vi "FP PC main.vi"() -> ()   [LabVIEW 2014]
panel:
  in  "Tab Control":enum32{"Front Page", "Mission Definition"}(tab)
  in  "Chase?":bool
  in  "stop":bool
  in  "Tug letter":string="T"
  out "UDP Time Out?":bool
  out "Blink":bool
  out "error IO":errorcluster
  out "GPS":cluster{"X pos":i32, "Y pos":i32, "Heading":dbl}
  out "Grid Image":T1(plugin-control)
  in  "Pool image\nfile name":string="leds in brightfield cropped.bmp"
  in  "Boat image\nfile name":string="large boat image.png"
  out "Occupancy Grid":u32[][](array[numeric])
  out "Buoy locations":cluster{"regular expression":string, i32, i32}[](array[cluster])
  out "GPS?":bool
  in  "Mission #":enum16{"1", "2", "3"}(ring)
  in  "Use mission?":bool
  in  "MDF Control":T2(array[cluster])=[{"Type"=enum."Start", "X"=100, "Y"=100, "Speed"=10, "Behaviors"=enum."Open Water Transit"}, {"Type"=enum."Waypoint", "X"=449, "Y"=569, "Speed"=4, "Behaviors"=enum."Open Water Transit"}, {"Type"=enum."Waypoint", "X"=803, "Y"=515, "Speed"=4, "Behaviors"=enum."Open Water Transit"}, {"Type"=enum."Waypoint", "X"=911, "Y"=689, "Speed"=4, "Behaviors"=enum."Open Water Transit"}, {"Type"=enum."Waypoint", "X"=755, "Y"=881, "Speed"=4, "Behaviors"=enum."Open Water Transit"}, {"Type"=enum."End", "X"=0, "Y"=0, "Speed"=0, "Behaviors"=enum."Open Water Transit"}]
  out "MDF To Send":T2(array[cluster])=[{"Type"=enum."Start", "X"=100, "Y"=100, "Speed"=10, "Behaviors"=enum."Open Water Transit"}, {"Type"=enum."Waypoint", "X"=449, "Y"=569, "Speed"=4, "Behaviors"=enum."Open Water Transit"}, {"Type"=enum."Waypoint", "X"=803, "Y"=515, "Speed"=4, "Behaviors"=enum."Open Water Transit"}, {"Type"=enum."Waypoint", "X"=911, "Y"=689, "Speed"=4, "Behaviors"=enum."Open Water Transit"}, {"Type"=enum."Waypoint", "X"=755, "Y"=881, "Speed"=4, "Behaviors"=enum."Open Water Transit"}, {"Type"=enum."End", "X"=0, "Y"=0, "Speed"=0, "Behaviors"=enum."Open Water Transit"}]
  # "This page is used to plan the mission.  The MDF, Mission Definition File, control below is used for that purpose.\n\n*  Each mission must begin with a record of type \"Start\" and end with a record of type \"End\"\n*  For the \"Start\" and \"End\" records the remaining entries have no impact.\n*  For the \"Waypoint\" records you must set a position for the waypoint, a speed, and a behavior.\n*  Any number of records may be used.\n*  The simulation will place a \"yellow\" marker at the local of each waypoint include.\n*  If you declare unused records type \"End\" they will not be include in the simulation"
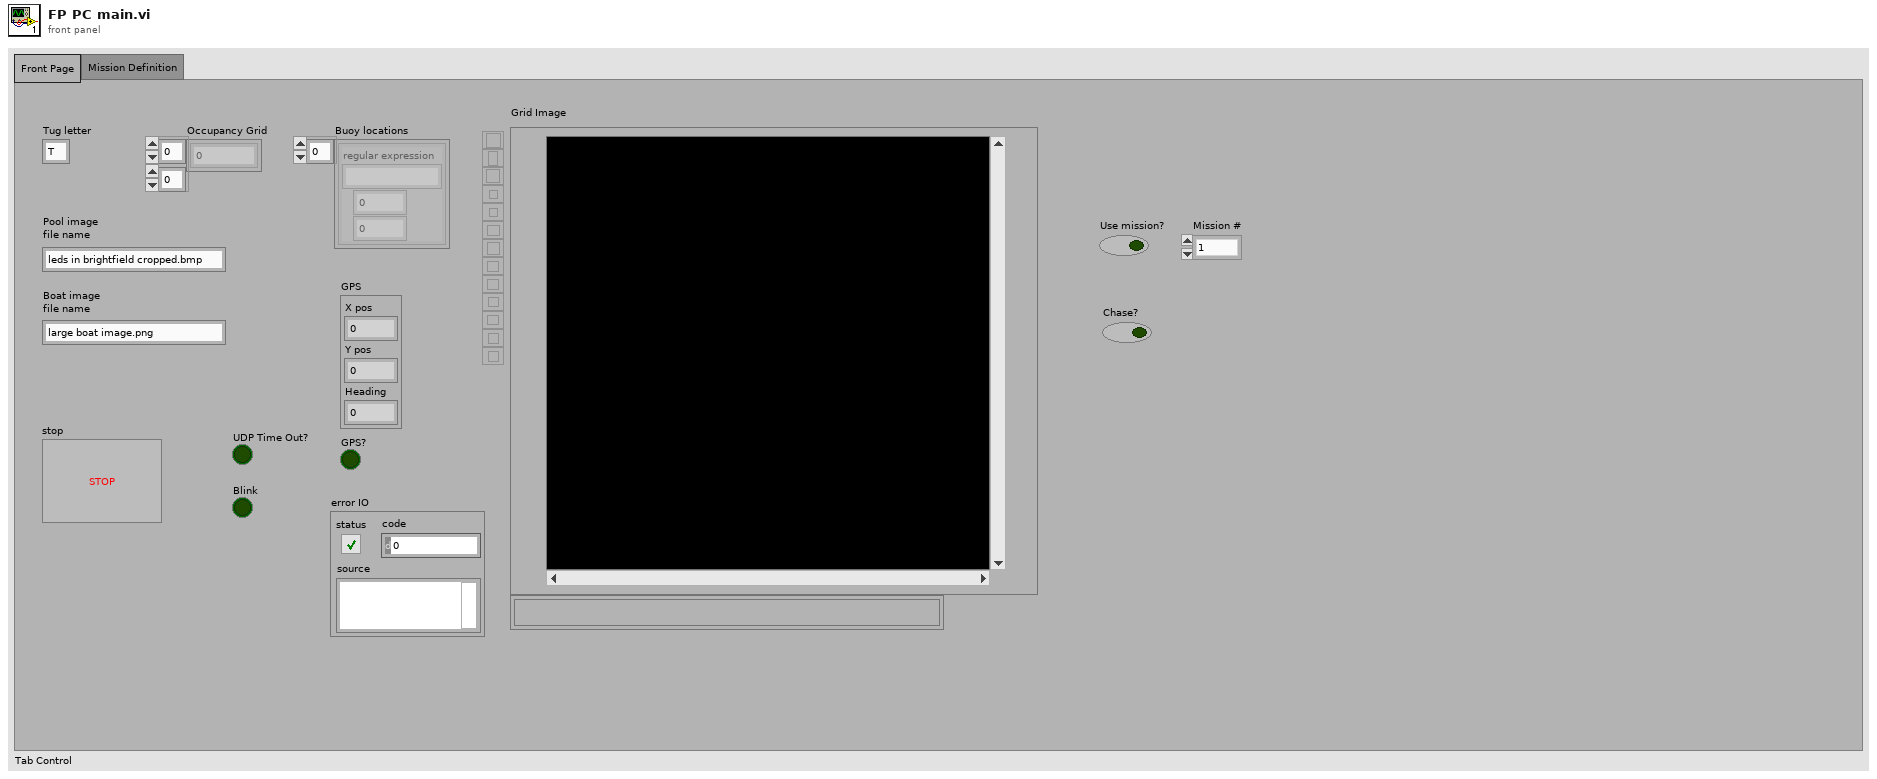
[diagram p1: front panel]
types:
  T1 = typedef "IMAQ Image.ctl" = refnum<image>
  T2 = cluster{"Type":enum16{"Start", "Waypoint", "End"}, "X":i32, "Y":i32, "Speed":i32, "Behaviors":enum16{"Open Water Transit", "P-Wall Follow", "S-Wall Follow", "Dock", "Chase"}}[]
  T3 = typedef "Image Type" = u32
  T4 = cluster{"regular expression":string, i32, i32, i32}
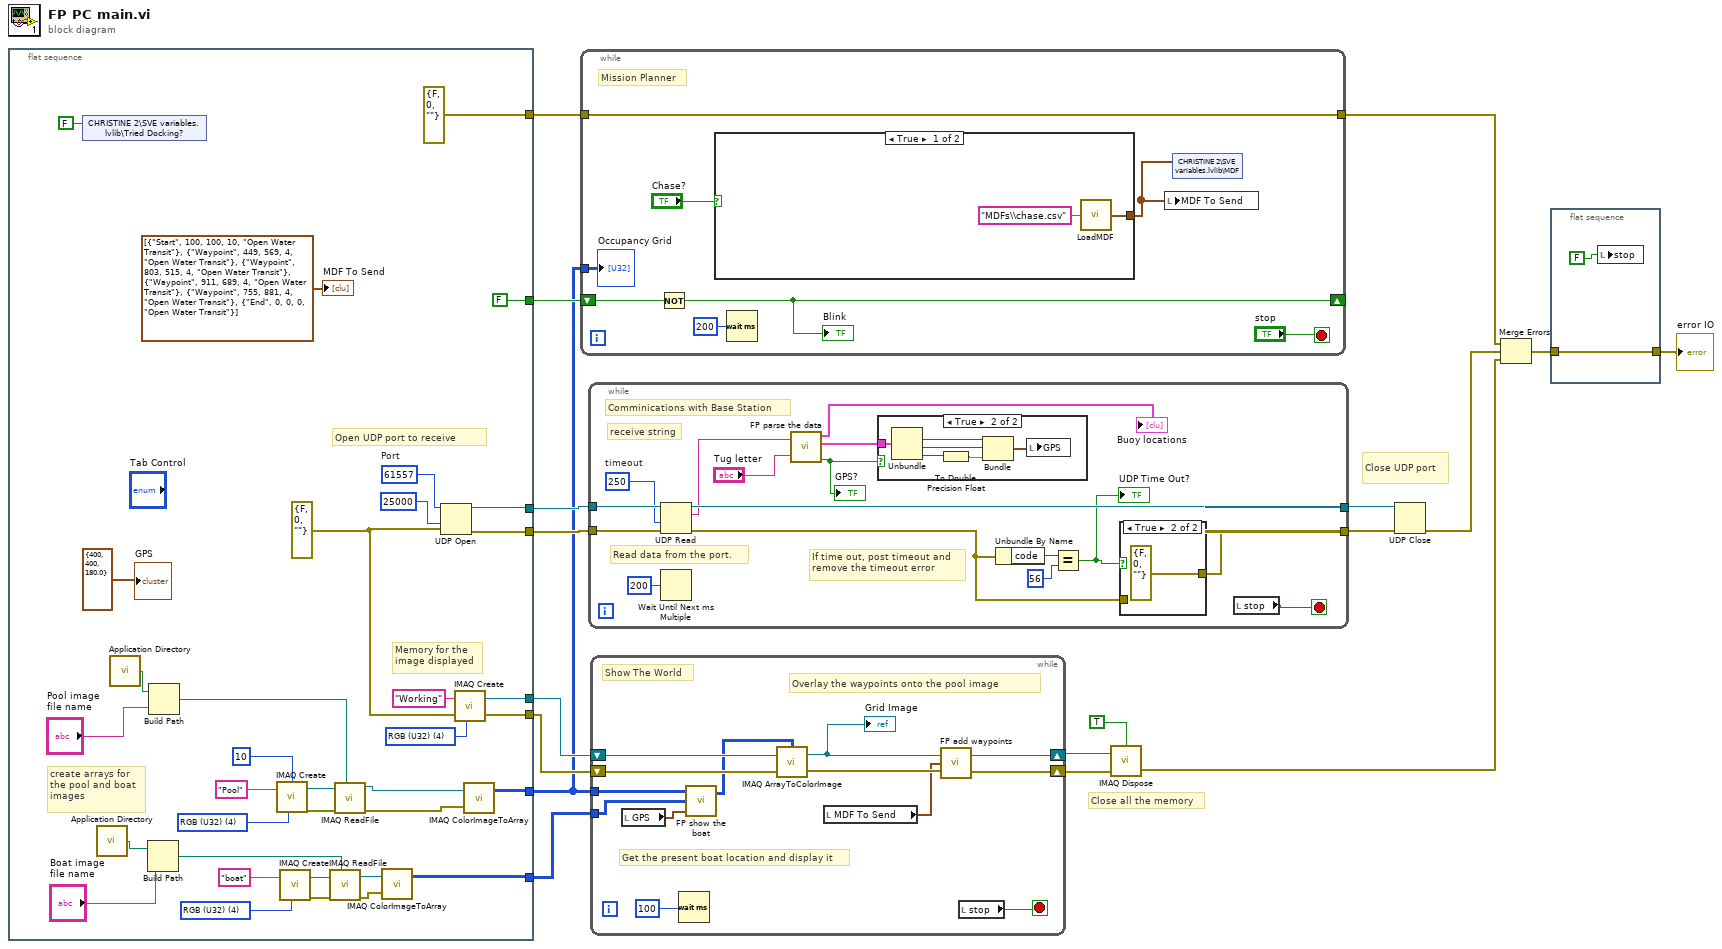
[diagram p0: block diagram]
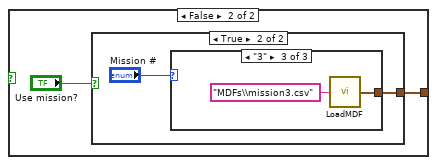
[diagram p4: hidden frame]
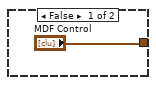
[diagram p5: hidden frame]
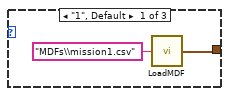
[diagram p6: hidden frame]
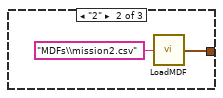
[diagram p7: hidden frame]
diagram:
  # "Close all the memory"
  # "Close UDP port"
  n1 = flat-sequence {
    tunnel: [errorcluster {"status"=FALSE, "code"=0, "source"=""} ("error in (no error)")] -> w18
    tunnel: [w50] -> w15
    tunnel: [w49] -> w14
    tunnel: [FALSE] -> w11
    tunnel: [w26] -> w7
    tunnel: [w25] -> w3
    tunnel: [w24] -> w6
    tunnel: [w23] -> w5
    frame #0 {
      w38 = T3 4 items=["Grayscale (U8)", "Grayscale (I16)", "Grayscale (SGL)", "Complex (CSG)", "RGB (U32)", "HSL (U32)", "RGB (U64)", "Grayscale (U16)"] ("Image Type")
      w34 = T3 4 items=["Grayscale (U8)", "Grayscale (I16)", "Grayscale (SGL)", "Complex (CSG)", "RGB (U32)", "HSL (U32)", "RGB (U64)", "Grayscale (U16)"] ("Image Type")
      w30 = T3 4 items=["Grayscale (U8)", "Grayscale (I16)", "Grayscale (SGL)", "Complex (CSG)", "RGB (U32)", "HSL (U32)", "RGB (U64)", "Grayscale (U16)"] ("Image Type")
      w22 = errorcluster {"status"=FALSE, "code"=0, "source"=""} ("error in (no error)")
      w51 = u16 61557  # Port
      # "Memory for the\nimage displayed"
      # "create arrays for\nthe pool and boat\nimages"
      # "Open UDP port to receive"
      n2 = shared-variable "CHRISTINE 2\\SVE variables.lvlib\\Tried Docking?"(FALSE ("Tried Docking?")) -> ()  [unwired: 1 in, 1 out]
      n3 = call <vilib>:"Application Directory.vi"() -> ("Application Directory"=w45:path)
      n4 = call <vilib>:"Application Directory.vi"() -> ("Application Directory"=w44:path)
      n5 = Build Path(base path=w45, name or relative path="Boat image\nfile name") -> (appended path=w47:path)
      n6 = Build Path(base path=w44, name or relative path="Pool image\nfile name") -> (appended path=w42:path)
      n7 = call "IMAQ Create"("Border Size"=10, "Image Name"="Pool", "Image Type"=w30) -> ("New Image"=w28:T1, "error out"=w29:errorcluster)  [unwired: 2 in]
      n8 = call "IMAQ Create"("Image Name"="boat", "Image Type"=w34) -> ("New Image"=w32:T1, "error out"=w33:errorcluster)  [unwired: 3 in]
      n9 = call "IMAQ ReadFile"("File Path"=w47, "error in (no error)"=w33, "Image"=w32) -> ("error out"=w36:errorcluster, "Image Out"=w37:T1)  [unwired: 4 in, 3 out]
      n10 = call "IMAQ ReadFile"("File Path"=w42, "error in (no error)"=w29, "Image"=w28) -> ("error out"=w41:errorcluster, "Image Out"=w40:T1)  [unwired: 4 in, 3 out]
      n11 = call "IMAQ ColorImageToArray"("Image"=w37, "error in (no error)"=w36) -> ("Image Pixels (U32)"=w26:u32[][])  [unwired: 2 in, 2 out]
      n12 = UDP Open(8:w22, 9:25000 ("timeout ms (25000)"), 11:w51) -> (port=w49:refnum<k16>, 0:w50:errorcluster)  [unwired: 2 in, 1 out]
      n13 = call "IMAQ Create"("Image Name"="Working", "Image Type"=w38, "error in (no error)"=w22) -> ("New Image"=w24:T1, "error out"=w23:errorcluster)  [unwired: 2 in]
      n14 = call "IMAQ ColorImageToArray"("Image"=w40, "error in (no error)"=w41) -> ("Image Pixels (U32)"=w25:u32[][])  [unwired: 2 in, 2 out]
      "GPS" <- cluster{i32, i32, dbl} {400, 400, 180.0} ("output cluster")
      "MDF To Send" <- T2 [{"Type"=enum."Start", "X"=100, "Y"=100, "Speed"=10, "Behaviors"=enum."Open Water Transit"}, {"Type"=enum."Waypoint", "X"=449, "Y"=569, "Speed"=4, "Behaviors"=enum."Open Water Transit"}, {"Type"=enum."Waypoint", "X"=803, "Y"=515, "Speed"=4, "Behaviors"=enum."Open Water Transit"}, {"Type"=enum."Waypoint", "X"=911, "Y"=689, "Speed"=4, "Behaviors"=enum."Open Water Transit"}, {"Type"=enum."Waypoint", "X"=755, "Y"=881, "Speed"=4, "Behaviors"=enum."Open Water Transit"}, {"Type"=enum."End", "X"=0, "Y"=0, "Speed"=0, "Behaviors"=enum."Open Water Transit"}] ("MDF To Send")
    }
  }
  n15 = while {
    tunnel: w18 -> [w59]
    tunnel: [w59] -> w12
    shift-right: [w57] -> _
    shift-left: w11 -> [w58]
    tunnel: w3 -> [w56]
    stop <- "stop" stop-if-true
    # "Mission Planner"
    n16 = Not(x=w58) -> (.not. x?=w57:bool)
    "Blink" <- w57
    n17 = case shown="True" "Chase?" {
      tunnel: [w62 w64] -> w55
      frame True {
        n18 = call "LoadMDF.vi"("relative path"="MDFs\\chase.csv") -> ("MDF"=w62:T2)
      }
      frame False {
        n19 = case shown="True" "Use mission?" {
          tunnel: ["MDF Control" w67] -> w64
          frame False {
          }
          frame True {
            n20 = case shown="\"3\"" "Mission #" {
              tunnel: [w69 w71 w73] -> w67
              frame "1", Default {
                n21 = call "LoadMDF.vi"("relative path"="MDFs\\mission1.csv") -> ("MDF"=w69:T2)
              }
              frame "2" {
                n22 = call "LoadMDF.vi"("relative path"="MDFs\\mission2.csv") -> ("MDF"=w71:T2)
              }
              frame "3" {
                n23 = call "LoadMDF.vi"("relative path"="MDFs\\mission3.csv") -> ("MDF"=w73:T2)
              }
            }
          }
        }
      }
    }
    n24 = Wait (ms)(milliseconds to wait=u32 200) -> ()  [unwired: 1 out]
    n25 = local write "MDF To Send"(w55) -> ()
    n26 = shared-variable "CHRISTINE 2\\SVE variables.lvlib\\MDF"(w55) -> ()  [unwired: 1 in, 1 out]
    "Occupancy Grid" <- w56
  }
  n27 = while {
    tunnel: w15 -> [w90]
    tunnel: w14 -> [w89]
    tunnel: [w88] -> w17
    tunnel: [w83] -> w16
    stop <- w80 stop-if-true
    w82 = 250  # timeout
    # "Comminications with Base Station"
    # "receive string"
    # "If time out, post timeout and\nremove the timeout error"
    # "Read data from the port."
    n28 = UDP Read(connection ID=w89, timeout ms (25000)=w82, 8:w90) -> (data out=w77:string, error out=w84:errorcluster, 3:w88:refnum<k16>)  [unwired: 1 in, 2 out]
    n29 = Wait Until Next ms Multiple(millisecond multiple=u32 200) -> ()  [unwired: 1 out]
    n30 = call "FP parse the data.vi"("Nav String"=w77, "Tug"="Tug letter") -> ("Buoy locations"=→"Buoy locations":cluster{"regular expression":string, i32, i32}[], "Tug Location"=w78:T4, "Valid?"=w75:bool)  [unwired: 1 out]
    "GPS?" <- w75
    n31 = case shown="True" w75 {
      tunnel: w78 -> [_ w96]
      frame False {
      }
      frame True {
        n32 = Unbundle(w96) -> (w95:i32, w94:i32, w92:i32)  [unwired: 1 out]
        n33 = To Double Precision Float(number=w92) -> (double precision float=w93:dbl)
        n34 = Bundle(w95, w94, w93) -> (w91:cluster{i32, i32, dbl})  [unwired: 1 in]
        n35 = local write "GPS"(w91) -> ()
      }
    }
    n36 = Unbundle By Name(w84) -> ("code"=w87:i32)
    n37 = Equal?(x=w87, y=56) -> (x = y?=w85:bool)
    "UDP Time Out?" <- w85
    n38 = case shown="True" w85 {
      tunnel: [w97 errorcluster {"status"=FALSE, "code"=0, "source"=""} ("error out")] -> w83
      tunnel: w84 -> [w97 _]
      frame False {
      }
      frame True {
      }
    }
    n39 = local read "stop"() -> (w80:bool)
  }
  n40 = while {
    tunnel: w7 -> [w103]
    tunnel: w3 -> [w104]
    shift-right: [w105] -> w9
    shift-left: w5 -> [w111]
    shift-right: [w106] -> w8
    shift-left: w6 -> [w110]
    stop <- w109 stop-if-true
    # "Overlay the waypoints onto the pool image"
    # "Show The World"
    # "Get the present boat location and display it"
    n41 = local read "GPS"() -> (w101:cluster{"X pos":i32, "Y pos":i32, "Heading":dbl})
    n42 = Wait (ms)(milliseconds to wait=u32 100) -> ()  [unwired: 1 out]
    n43 = call "FP show the boat.vi"("GPS"=w101, "Boat array"=w103, "Pool array"=w104) -> ("Pool out"=w100:u32[][])  [unwired: 1 in]
    n44 = call "IMAQ ArrayToColorImage"("Image Pixels (U32)"=w100, "Image"=w110, "error in (no error)"=w111) -> ("Image Out"=w107:T1, "error out"=w108:errorcluster)  [unwired: 2 in]
    "Grid Image" <- w107
    n45 = local read "MDF To Send"() -> (w99:T2)
    n46 = call "FP add waypoints.vi"("error in"=w108, "MDF Control"=w99, "Image In"=w107) -> ("error out"=w105:errorcluster, "Image Out"=w106:T1)
    n47 = local read "stop"() -> (w109:bool)
  }
  n48 = call "IMAQ Dispose"("All Images? (No)"=TRUE, "Image"=w8, "error in (no error)"=w9) -> ("error out"=w4:errorcluster)  [unwired: 3 in]
  n49 = UDP Close(connection ID=w17, 8:w16) -> (error out=w13:errorcluster)  [unwired: 1 out]
  n50 = Merge Errors(w12, w13, w4) -> (w1:errorcluster)
  n51 = flat-sequence {
    tunnel: [w113] -> w2
    tunnel: w1 -> [w113]
    frame #0 {
      n52 = local write "stop"(FALSE) -> ()
    }
  }
  "error IO" <- w2
